vi "Read Attribute Data.vi"(8 "error in (no error)":errorcluster, 10 "Object Name":string, 11 "CS++Factory in":refnum<class "CS++Factory.lvclass">) -> (0 "error out":errorcluster, 2 "Attribute Data":variant, 3 "CS++Factory out":refnum<class "CS++Factory.lvclass">)   [LabVIEW 2015, in "CS++BaseClasses.lvlib" / "CS++Factory.lvclass"]
doc: "Read object attribute data from storage medium.\n\nThe default implementation reads from ini-file."
uses:
  CS++Factory.lvclass
  CS++Factory.lvclass/CS++Factory.ctl
  <vilib>/Utility/config.llb/Read Key (String).vi
  <vilib>/Utility/config.llb/NI_LVConfig.lvlib
  Libraries/Utilities/CS++Utilities.lvlib
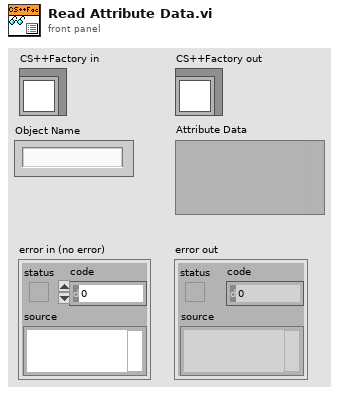
[diagram p1: front panel]
types:
  T1 = typedef "NI_LVConfig.lvlib/Config Data RefNum.ctl" = refnum<k1>
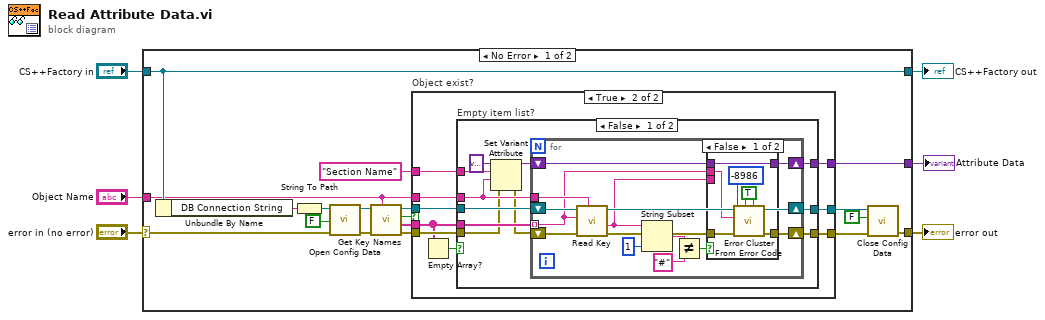
[diagram p0: block diagram]
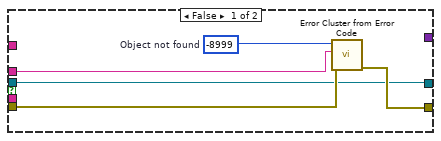
[diagram p2: hidden frame]
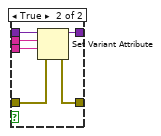
[diagram p3: hidden frame]
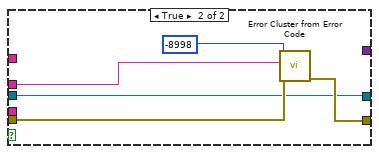
[diagram p4: hidden frame]
diagram:
  n1 = case shown="No Error" "error in (no error)" {
    selector: "error in (no error)" -> [w15 w82]
    tunnel: [w14 w82] -> w5
    tunnel: [w24 w81] -> w3
    tunnel: "CS++Factory in" -> [w24 w81]
    tunnel: [w13 _] -> w2
    tunnel: "Object Name" -> [w12 _]
    frame No Error {
      n2 = Unbundle By Name(w24) -> ("DB Connection String"=w7:string)
      n3 = String To Path(string=w7) -> (path=w8:path)
      n4 = call <vilib>:"Open Config Data.vi"("error in (no error)"=w15, "create file if necessary (T)"=FALSE, "configuration file path"=w8) -> ("error out"=w18:errorcluster, "refnum"=w19:T1)  [unwired: 6 in, 1 out]
      n5 = call <vilib>:"Get Key Names.vi"("section"=w12, "error in (no error)"=w18, "refnum"=w19) -> ("error out"=w17:errorcluster, "key names"=w11:string[], "section exists?"=w10:bool, "refnum out"=w16:T1)  [unwired: 5 in]
      n6 = case "Object exist?" shown="True" w10 {
        tunnel: "Section Name" ("name") -> [_ w38]
        tunnel: [w26 w37] -> w22
        tunnel: [w27 w36] -> w21
        tunnel: w17 -> [w28 w35]
        tunnel: w16 -> [w26 w34]
        tunnel: [_ w33] -> w13
        tunnel: w12 -> [w25 w32]
        tunnel: w11 -> [_ w31]
        frame False {
          w29 = -8999  # Object not found
          n7 = call <vilib>:"Error Cluster from Error Code.vi"("Error In"=w28, "Error Message (\"\")"=w25, "Error Code (0)"=w29) -> ("Error Out"=w27:errorcluster)  [unwired: 8 in]
        }
        frame True {
          n8 = Empty Array?(array=w31) -> (empty?=w30:bool)
          n9 = case "Empty item list?" shown="False" w30 {
            tunnel: w38 -> [w42 _]
            tunnel: [w49 w76] -> w37
            tunnel: [w48 w79] -> w36
            tunnel: w35 -> [w40 w80]
            tunnel: w34 -> [w47 w76]
            tunnel: w31 -> [w46 _]
            tunnel: [w45 _] -> w33
            tunnel: w32 -> [w41 w77]
            frame False {
              n10 = Set Variant Attribute(Variant=variant ("variant"), name=w42, value=w41, error in=w40) -> (Variant out=w43:variant, error out=w39:errorcluster)  [unwired: 1 out]
              n11 = for {
                tunnel: w46 -> [w59] mode=indexing
                tunnel: w41 -> [w61]
                shift-right: [w57] -> w48
                shift-left: w39 -> [w62]
                shift-right: [w56] -> w45
                shift-left: w43 -> [w60]
                shift-right: [w55] -> w49
                shift-left: w47 -> [w63]
                n12 = call-poly <vilib>:"Read Key.vi"("section"=w61, "error in (no error)"=w62, "key"=w59, "refnum"=w63) -> ("error out"=w58:errorcluster, "value"=w54:string, "refnum out"=w55:T1)  [unwired: 4 in, 1 out]
                n13 = String Subset(string=w54, length (rest)=1 ("length (rest)")) -> (substring=w52:string)  [unwired: 1 in]
                n14 = Not Equal?(x=w52, y="#") -> (x != y?=w50:bool)
                n15 = case shown="False" w50 {
                  tunnel: w60 -> [w69 w75]
                  tunnel: w59 -> [w65 w74]
                  tunnel: w54 -> [_ w73]
                  tunnel: w58 -> [w68 w72]
                  tunnel: [w67 w71] -> w57
                  tunnel: [w69 w70] -> w56
                  frame False {
                    w64 = TRUE ("is warning? (False)")
                    n16 = call <vilib>:"Error Cluster From Error Code.vi"("is warning? (False)"=w64, "show call chain? (False)"=w64, "error in (no error)"=w68, "error message (\"\")"=w65, "error code (0)"=-8986) -> ("error out"=w67:errorcluster)  [unwired: 4 in]
                  }
                  frame True {
                    n17 = Set Variant Attribute(Variant=w75, name=w74, value=w73, error in=w72) -> (Variant out=w70:variant, error out=w71:errorcluster)  [unwired: 1 out]
                  }
                }
              }
            }
            frame True {
              n18 = call <vilib>:"Error Cluster from Error Code.vi"("Error In"=w80, "Error Message (\"\")"=w77, "Error Code (0)"=-8998 ("Object configuration data not found")) -> ("Error Out"=w79:errorcluster)  [unwired: 8 in]
            }
          }
        }
      }
      n19 = call <vilib>:"Close Config Data.vi"("error in (no error)"=w21, "write file if changed (T)"=FALSE, "refnum"=w22) -> ("error out"=w14:errorcluster)  [unwired: 7 in, 1 out]
    }
    frame Error {
    }
  }
  "error out" <- w5
  "CS++Factory out" <- w3
  "Attribute Data" <- w2
